vi "Global senso rotazione.vi"() -> ()   [LabVIEW 2019]
panel:
  out "Senso rot (T<0 F>0)":bool
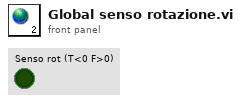
[diagram p1: front panel]
diagram:
